vi "Update Value.vi"(6 "Time":dbl, 8 "error in (no error)":errorcluster, 11 "GaugeIndicator in":refnum<class "GaugeIndicator.lvclass">) -> (0 "error out":errorcluster, 1 "Update":bool, 2 "Value":variant, 3 "GaugeIndicator out":refnum<class "GaugeIndicator.lvclass">)   [LabVIEW 2020, in "VolatusGUIElements.lvlib" / "GaugeIndicator.lvclass"]
uses:
  GaugeIndicator.lvclass
  GaugeIndicator.lvclass/GaugeIndicator.ctl
  lv-vecto/Vecto/Channel/Channel.lvclass/Channel.ctl
  lv-vecto/Vecto/Group/Value by Index.vi
  lv-vecto/Vecto/Channel/Channel.lvclass
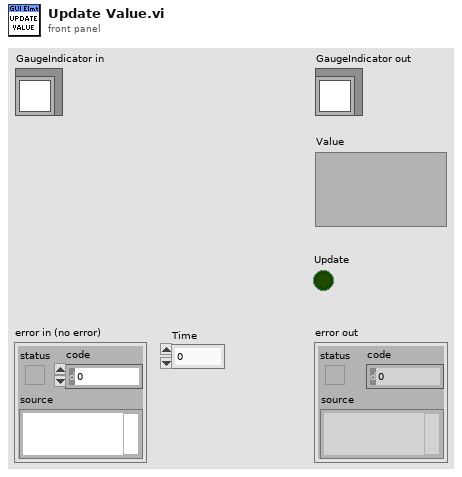
[diagram p1: front panel]
types:
  T1 = typedef "VolatusGUIElements.lvlib/GaugeIndicator.lvclass/Value Source.ctl" = enum16{"Constant", "Channel"}
  T2 = cluster{"Color Band":picture, "Scaled":dbl, "Max":dbl, "Min":dbl}
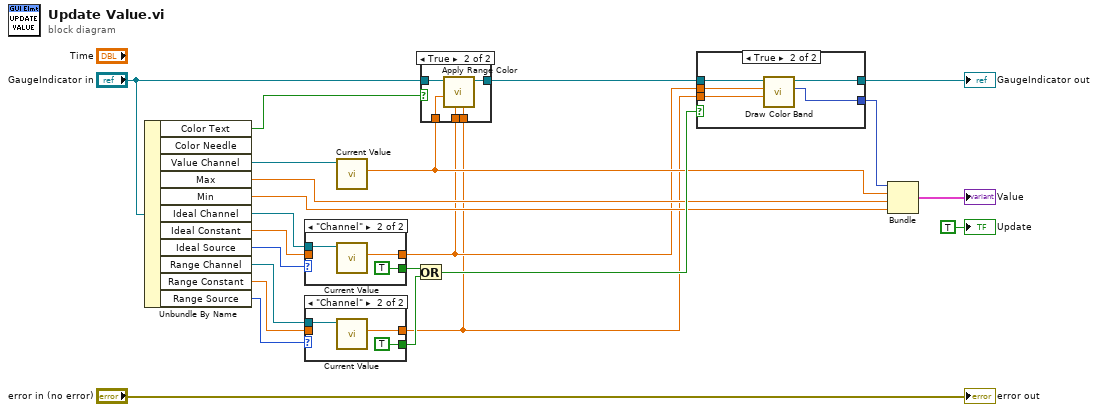
[diagram p0: block diagram]
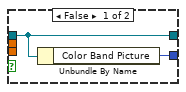
[diagram p3: hidden frame]
diagram:
  n1 = Unbundle By Name("GaugeIndicator in") -> ("Color Text"=w4:bool, "Value Channel"=w16:refnum<class "Channel.lvclass">, "Max"=w10:dbl, "Min"=w11:dbl, "Ideal Channel"=w19:refnum<class "Channel.lvclass">, "Ideal Constant"=w18:dbl, "Ideal Source"=w17:T1, "Range Channel"=w21:refnum<class "Channel.lvclass">, "Range Constant"=w20:dbl, "Range Source"=w22:T1)  [unwired: 1 out]
  n2 = case shown="\"Channel\"" w17 {
    tunnel: w19 -> [_ w27]
    tunnel: w18 -> [w24 _]
    tunnel: [w24 w26] -> w2
    tunnel: [_ TRUE] -> w15
    frame "Constant" {
    }
    frame "Channel" {
      n3 = call "Current Value.vi"("Channel in"=w27) -> ("Scaled"=w26:dbl)  [unwired: 6 in, 4 out]
    }
  }
  n4 = case shown="\"Channel\"" w22 {
    tunnel: w21 -> [_ w31]
    tunnel: w20 -> [w28 _]
    tunnel: [w28 w30] -> w1
    tunnel: [_ TRUE] -> w14
    frame "Constant" {
    }
    frame "Channel" {
      n5 = call "Current Value.vi"("Channel in"=w31) -> ("Scaled"=w30:dbl)  [unwired: 6 in, 4 out]
    }
  }
  n6 = call "Current Value.vi"("Channel in"=w16) -> ("Scaled"=w3:dbl)  [unwired: 6 in, 4 out]
  n7 = Or(x=w15, y=w14) -> (x .or. y?=w13:bool)
  n8 = case shown="True" w4 {
    tunnel: "GaugeIndicator in" -> [w32 w37]
    tunnel: [w32 w36] -> w5
    tunnel: w3 -> [_ w35]
    tunnel: w2 -> [_ w34]
    tunnel: w1 -> [_ w33]
    frame False {
    }
    frame True {
      n9 = call "Apply Range Color.vi"("Range"=w33, "Ideal"=w34, "Value"=w35, "GaugeIndicator in"=w37) -> ("GaugeIndicator out"=w36:refnum<class "GaugeIndicator.lvclass">)  [unwired: 6 in, 1 out]
    }
  }
  n10 = case shown="True" w13 {
    tunnel: w5 -> [w39 w44]
    tunnel: w2 -> [_ w43]
    tunnel: w1 -> [_ w42]
    tunnel: [w39 w40] -> w7
    tunnel: [w38 w41] -> w12
    frame False {
      n11 = Unbundle By Name(w39) -> ("Color Band Picture"=w38:picture)
    }
    frame True {
      n12 = call "Draw Color Band.vi"("Range"=w42, "Ideal"=w43, "GaugeIndicator in"=w44) -> ("Color Band"=w41:picture, "GaugeIndicator out"=w40:refnum<class "GaugeIndicator.lvclass">)  [unwired: 6 in, 1 out]
    }
  }
  "GaugeIndicator out" <- w7
  n13 = Bundle("Color Band"=w12, "Scaled"=w3, "Max"=w10, "Min"=w11) -> (→"Value":T2)  [unwired: 1 in]
  "error out" <- "error in (no error)"
  "Update" <- TRUE ("Update")
